vi "input.vi"(8 "error in":errorcluster, 10 "data table in":T1, 11 "tag bus configurable plugin module in":refnum<class "tag bus configurable plugin module.lvclass">) -> (0 "error out":errorcluster, 2 "data table out":T1, 3 "tag bus configurable plugin module out":refnum<class "tag bus configurable plugin module.lvclass">)   [LabVIEW 2014, in "tag bus configurable plugin module.lvclass"]
doc: "Provides an interface for reading data from a module at runtime. While this interface performs no operations, a child should provide an override which may read from any open sessions, references, or interfaces."
uses:
  tag bus configurable plugin module.lvclass
  <vilib>/NI/Tag Bus/table/data table.ctl
  <vilib>/NI/Tag Bus/table/data polymorphs/write one/write Double.vi
  <vilib>/NI/Tag Bus/table/data table.lvlib
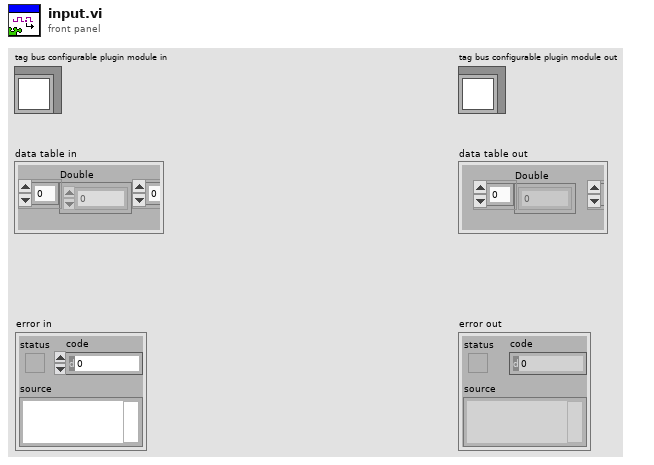
[diagram p1: front panel]
types:
  T1 = typedef "tag bus.lvlib/data table.lvlib/data table.ctl" = cluster{"Double":dbl[], "Single":sgl[], "I64":i64[], "I32":i32[], "I16":i16[], "I8":i8[], "U64":u64[], "U32":u32[], "U16":u16[], "U8":u8[], "Boolean":bool[], "String":string[], "Array of Double":cluster{"DBL Array":dbl[]}[], "Array of Single":cluster{"SGL Array":sgl[]}[], "Array of I64":cluster{"I64 Array":i64[]}[], "Array of I32":cluster{"I32 Array":i32[]}[], "Array of I16":cluster{"I16 Array":i16[]}[], "Array of I8":cluster{"I8 Array":i8[]}[], "Array of U64":cluster{"U64 Array":u64[]}[], "Array of U32":cluster{"U32 Array":u32[]}[], "Array of U16":cluster{"U16 Array":u16[]}[], "Array of U8":cluster{"U8 Array":u8[]}[], "Array of Boolean":cluster{"Boolean Array":bool[]}[], "Array of String":cluster{"String Array":string[]}[]}
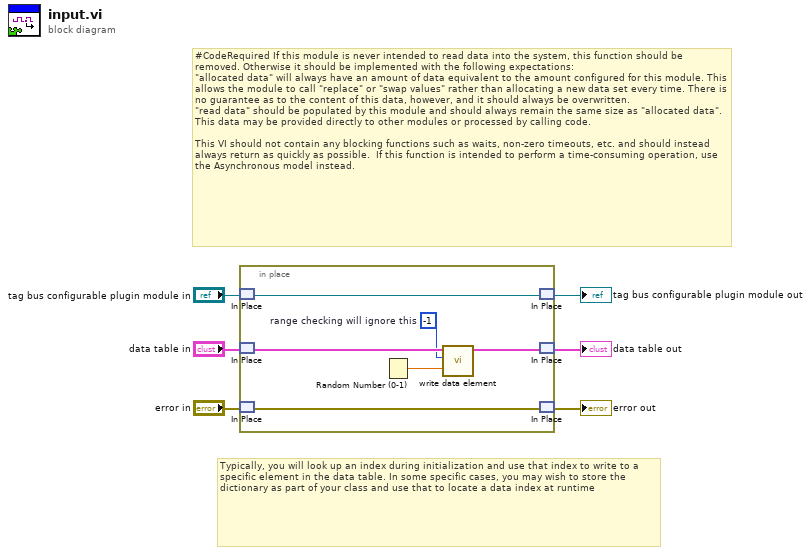
[diagram p0: block diagram]
diagram:
  # "Typically, you will look up an index during initialization and use that index to write to a specific element in the data table. In some specific cases, you may wish to store the dictionary as part of your class and use that to locate a data index at runtime"
  # "#CodeRequired If this module is never intended to read data into the system, this function should be removed. Otherwise it should be implemented with the following expectations:\n\"allocated data\" will always have an amount of data equivalent to the amount configured for this module. This allows the module to call \"replace\" or \"swap values\" rather than allocating a new data set every time. There is no guarantee as to the content of this data, however, and it should always be overwritten.\n\"read data\" should be populated by this module and should always remain the same size as \"allocated data\". This data may be provided directly to other modules or processed by calling code.\n\nThis VI should not contain any blocking functions such as waits, non-zero timeouts, etc. and should instead always return as quickly as possible.  If this function is intended to perform a time-consuming operation, use the Asynchronous model instead."
  n1 = in-place {
    w8 = -1  # range checking will ignore this
    n2 = in-place-match #1("tag bus configurable plugin module in") -> (w11:refnum<class "tag bus configurable plugin module.lvclass">)
    n3 = in-place-match #2("data table in") -> (w10:T1)
    n4 = in-place-match #3("error in") -> (w12:errorcluster)
    n5 = Random Number (0-1)() -> (number: 0 to 1=w7:dbl)
    n6 = call-poly <vilib>:"write data element.vi"("value"=w7, "index"=w8, "data table in"=w10) -> ("data table out"=w9:T1)  [unwired: 8 in]
    n7 = in-place-match #1(w11) -> (→"tag bus configurable plugin module out":refnum<class "tag bus configurable plugin module.lvclass">)
    n8 = in-place-match #2(w9) -> (→"data table out":T1)
    n9 = in-place-match #3(w12) -> (→"error out":errorcluster)
  }
